vi "publish.vi"(8 "error in":errorcluster, 9 "timeout":i32, 10 "stream definition":T1, 11 "stream publisher in":refnum<class "publisher.lvclass">) -> (0 "error out":errorcluster, 1 "timed out?":bool, 3 "stream publisher out":refnum<class "publisher.lvclass">)   [LabVIEW 2013, in "data stream.lvlib" / "publisher.lvclass"]
uses:
  publisher.lvclass
  stream definition.ctl
  message definition.ctl
  publisher.lvclass/publisher.ctl
  subscriber/subscriber.lvclass
  subscriber/subscriber.lvclass/subscriber.ctl
  data stream.lvlib
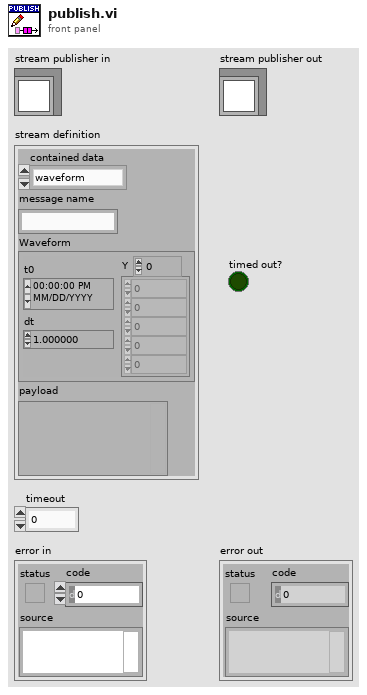
[diagram p1: front panel]
types:
  T1 = typedef "data stream.lvlib/stream definition.ctl" = cluster{"contained data":T2, "message name":string, "Waveform":waveform(dbl), "payload":variant}
  T2 = typedef "data stream.lvlib/message definition.ctl" = enum16{"waveform", "message"}
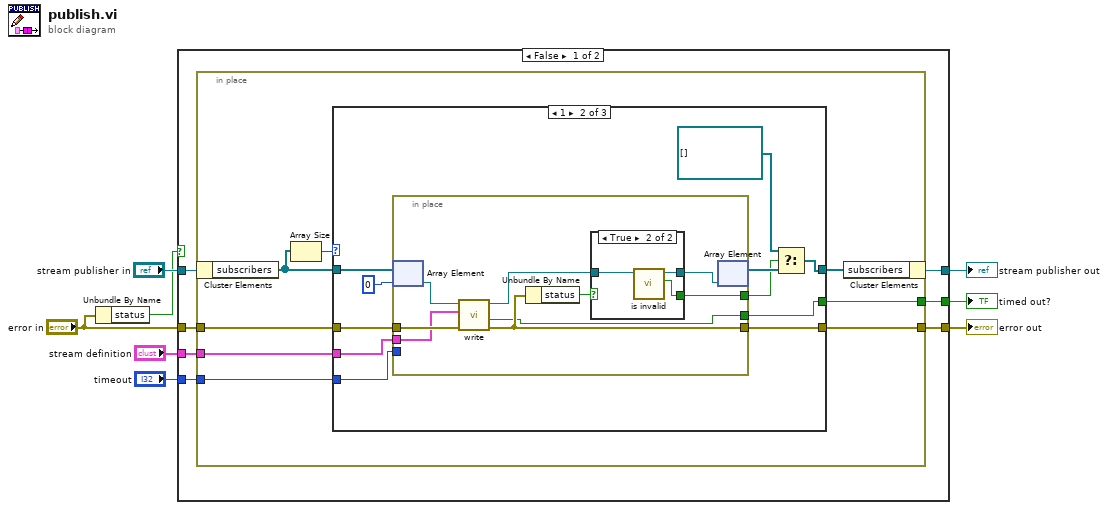
[diagram p0: block diagram]
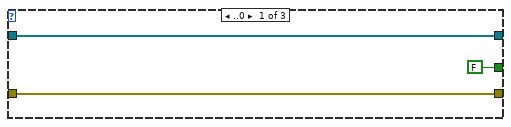
[diagram p2: hidden frame]
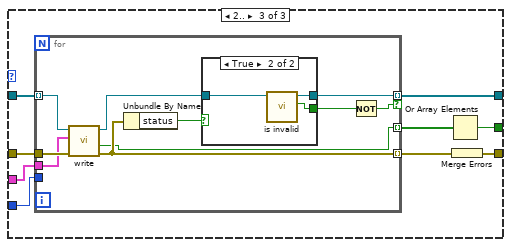
[diagram p4: hidden frame]
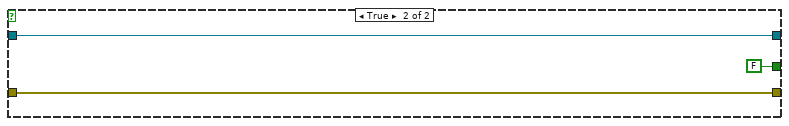
[diagram p6: hidden frame]
diagram:
  n1 = Unbundle By Name("error in") -> ("status"=w2:bool)
  n2 = case shown="False" w2 {
    tunnel: "stream publisher in" -> [w15 w76]
    tunnel: "timeout" -> [w14 _]
    tunnel: "error in" -> [w13 w75]
    tunnel: "stream definition" -> [w12 _]
    tunnel: [w11 w75] -> w5
    tunnel: [w10 w76] -> w4
    tunnel: [w9 FALSE ("timed out?")] -> w1
    frame False {
      n3 = in-place {
        in-place-border: w14 -> [w22]
        in-place-border: w13 -> [w21]
        in-place-border: [w20] -> w11
        in-place-border: w12 -> [w19]
        in-place-border: [w17] -> w9
        n4 = in-place-cluster #1(w15) -> ("subscribers"=w23:refnum<class "subscriber.lvclass">[])
        n5 = Array Size(array=w23) -> (size(s)=w16:i32)
        n6 = case shown="1" w16 {
          tunnel: [w26 w32 w53] -> w18
          tunnel: w23 -> [w26 w36 w57]
          tunnel: w21 -> [w25 w37 w59]
          tunnel: [w25 w28 w54] -> w20
          tunnel: w19 -> [_ w34 w56]
          tunnel: w22 -> [_ w33 w55]
          tunnel: [FALSE ("timed out?") w27 w51] -> w17
          frame ..0 {
          }
          frame 1 {
            n7 = in-place {
              in-place-border: w37 -> [w46]
              in-place-border: [w41] -> w28
              in-place-border: w34 -> [w44]
              in-place-border: w33 -> [_]
              in-place-border: [w40] -> w29
              in-place-border: [w38] -> w27
              n8 = in-place-array #2(w36, 0) -> (w45:refnum<class "subscriber.lvclass">)
              n9 = call "write.vi"("error in"=w46, "element"=w44, "stream publisher in"=w45) -> ("error out"=w41:errorcluster, "timed out?"=w38:bool, "stream publisher out"=w42:refnum<class "subscriber.lvclass">)  [unwired: 6 in]
              n10 = Unbundle By Name(w41) -> ("status"=w39:bool)
              n11 = case shown="True" w39 {
                tunnel: [w47 w49] -> w43
                tunnel: w42 -> [w47 w50]
                tunnel: [_ w48] -> w40
                frame False {
                }
                frame True {
                  n12 = call "is invalid.vi"("stream publisher in"=w50) -> ("invalid?"=w48:bool, "stream publisher out"=w49:refnum<class "subscriber.lvclass">)  [unwired: 9 in]
                }
              }
              n13 = in-place-array #2(w43) -> (w31:refnum<class "subscriber.lvclass">[])  [unwired: 1 out]
            }
            n14 = Select(t=refnum<class "subscriber.lvclass">[] [], s=w29, f=w31) -> (s? t:f=w32:refnum<class "subscriber.lvclass">[])
          }
          frame 2.. {
            n15 = for {
              tunnel: w59 -> [w69]
              tunnel: [w68] -> w58 mode=indexing
              tunnel: w57 -> [w64] mode=indexing
              tunnel: w56 -> [w67]
              tunnel: w55 -> [_]
              tunnel: [w63] -> w53 mode=indexing if=w62
              tunnel: [w60] -> w52 mode=indexing
              n16 = call "write.vi"("error in"=w69, "element"=w67, "stream publisher in"=w64) -> ("error out"=w68:errorcluster, "timed out?"=w60:bool, "stream publisher out"=w65:refnum<class "subscriber.lvclass">)  [unwired: 6 in]
              n17 = Unbundle By Name(w68) -> ("status"=w61:bool)
              n18 = case shown="True" w61 {
                tunnel: [w70 w72] -> w63
                tunnel: w65 -> [w70 w73]
                tunnel: [_ w71] -> w66
                frame False {
                }
                frame True {
                  n19 = call "is invalid.vi"("stream publisher in"=w73) -> ("invalid?"=w71:bool, "stream publisher out"=w72:refnum<class "subscriber.lvclass">)  [unwired: 9 in]
                }
              }
              n20 = Not(x=w66) -> (.not. x?=w62:bool)
            }
            n21 = Or Array Elements(Boolean array=w52) -> (logical OR=w51:bool)
            n22 = Merge Errors(w58) -> (w54:errorcluster)
          }
        }
        n23 = in-place-cluster #1("subscribers"=w18) -> (w10:refnum<class "publisher.lvclass">)
      }
    }
    frame True {
    }
  }
  "error out" <- w5
  "stream publisher out" <- w4
  "timed out?" <- w1
